vi "die.vi"(6 "timeout in ms (-1)":i32=-1, 7 "references":T1, 8 "error in (no error)":errorcluster) -> (0 "error out":errorcluster)   [LabVIEW 2015, in "repub-dvr_nre.lvlib"]
doc: "This VI will enqueue a command to the input queue which will cause the main loop to stop. It will also write a true to the stop notifier. By default the timeout is -1 (wait forever). In the event that a non negative timeout is provided it will output an error if a timeout occurs."
uses:
  repub-dvr_nre.lvlib
  public/_controls/references.ctl
  _controls/input.ctl
  _controls/input_command.ctl
  _controls/output.ctl
  _controls/data.ctl
  public/_controls/configuration.ctl
  lv-recipe-machine/private/_controls/recipe_data.ctl
  lv-recipe-machine/public/_controls/mode.ctl
  lv-recipe-machine/public/_controls/manual_state.ctl
  lv-recipe-machine/public/_controls/automatic_state.ctl
  <userlib>/antonio-alexander/lv-waitgroup/public/_controls/api_waitgroup.ctl
  lv-recipe-machine/public/_controls/transition.ctl
  public/_controls/change.ctl
  public/_controls/status.ctl
  public/_controls/error.ctl
  lv-recipe-machine/lv-recipe-machine.lvlib
  <userlib>/antonio-alexander/lv-waitgroup/lv-waitgroup.lvlib
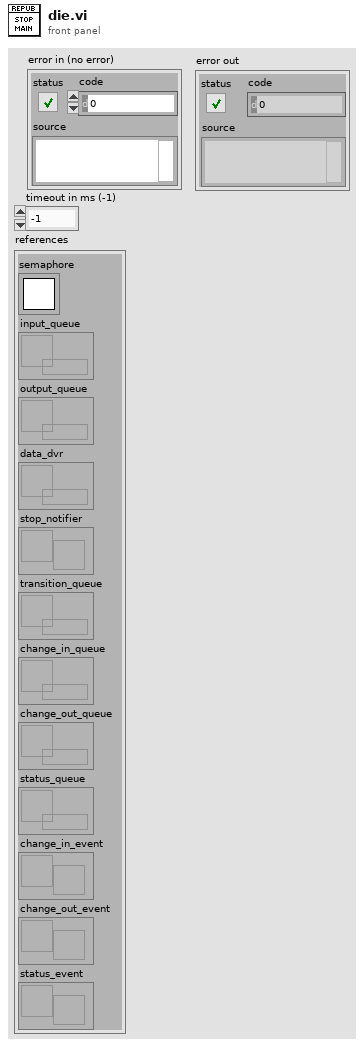
[diagram p1: front panel]
types:
  T1 = typedef "repub-dvr_nre.lvlib/references.ctl" = cluster{"semaphore":T2, "input_queue":refnum<queue>, "output_queue":refnum<queue>, "data_dvr":refnum<data-value>, "stop_notifier":refnum<notifier>, "transition_queue":refnum<queue>, "change_in_queue":refnum<queue>, "change_out_queue":refnum<queue>, "status_queue":refnum<queue>, "change_in_event":refnum<user-event>, "change_out_event":refnum<user-event>, "status_event":refnum<user-event>}
  T2 = typedef "Semaphore RefNum" = refnum<k1>
  T3 = typedef "repub-dvr_nre.lvlib/input.ctl" = cluster{"command":T4, "data":variant}
  T4 = typedef "repub-dvr_nre.lvlib/input_command.ctl" = enum8{"<input_command>", "die", "<null>"}
  T5 = typedef "repub-dvr_nre.lvlib/error.ctl" = enum16{"<error>", "bad_command", "command_queue_timeout", "stop_notifier_timeout", "die_command_timeout", "<null>"}
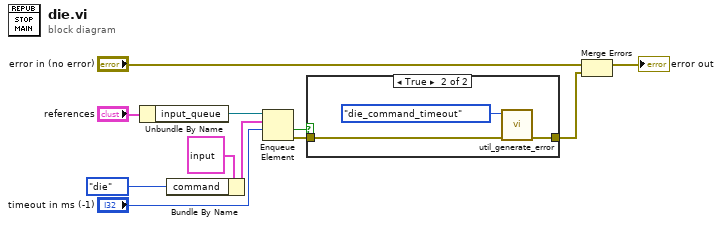
[diagram p0: block diagram]
diagram:
  n1 = Unbundle By Name("references") -> ("input_queue"=w11:refnum<queue>)
  n2 = Bundle By Name(cluster=T3 {"command"=enum."<input_command>", "data"=variant(cluster{"data":variant} {"data"=variant})} ("input"), "command"=input_command."die") -> (w1:T3)
  n3 = Enqueue Element(queue=w11, element=w1, timeout in ms (-1)="timeout in ms (-1)") -> (timed out?=w4:bool, error out=w6:errorcluster)  [unwired: 1 in, 1 out]
  n4 = case shown="True" w4 {
    tunnel: w6 -> [w12 w14]
    tunnel: [w12 w13] -> w5
    frame False {
    }
    frame True {
      n5 = call "util_generate_error.vi"("error in (no error)"=w14, "error"=error."die_command_timeout") -> ("error out"=w13:errorcluster)  [unwired: 9 in]
    }
  }
  n6 = Merge Errors("error in (no error)", w5) -> (→"error out":errorcluster)
